vi "Point Turn.vi"(9 "Speed":dbl, 10 "Angle":dbl) -> ()   [LabVIEW 2019]
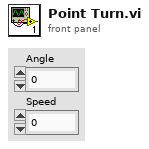
[diagram p1: front panel]
types:
  T1 = typedef "WPI_EncoderDevRef.ctl" = cluster{"DevStatus":errorcluster, "EncoderIndex":T2, "CounterIndex":T3, "DistancePerCount":dbl, "Decoding Type":T4}
  T2 = typedef "FPGA_EncoderIdx.ctl" = enum8{"Enc 0", "Enc 1", "Enc 2", "Enc 3", "Enc 4", "Enc 5", "Enc 6", "Enc 7", "Invalid"}
  T3 = typedef "FPGA_CounterCtrSystemIndex.ctl" = enum8{"Ctr 0", "Ctr 1", "Ctr 2", "Ctr 3", "Ctr 4", "Ctr 5", "Ctr 6", "Ctr 7", "Invalid"}
  T4 = typedef "WPI_EncoderType.ctl" = enum16{"1x", "2x", "4x"}
  T5 = typedef "WPI_RobotDriveDevRef.ctl" = cluster{"DevStatus":errorcluster, "Motors[]":T6[], "Square Inputs":bool, "Max Output":dbl}
  T6 = typedef "WPI_MotorControlDeviceRef.ctl" = cluster{"DeviceStatus":errorcluster, "Type":T7, "PWM":cluster{"PWM Channel":T8, "DeadBand":T9}, "CAN":cluster{"Device Number":u8, "SetOutput VI Ref":variant, "GetOutput VI Ref":variant, "Enable VI Ref":variant, "Disable VI Ref":variant, "Data":variant}, "Invert":bool, "DIO PWM":cluster{"PWM \"Enable\" Channel":T8, "DIOChannel":T10, "PWM Rate":dbl}}
  T7 = typedef "WPI_MotorControlType.ctl" = enum16{"PWM", "CAN", "DIO PWM"}
  T8 = typedef "FPGA_DIOPWMChannel.ctl" = enum8{"PWM 0", "PWM 1", "PWM 2", "PWM 3", "PWM 4", "PWM 5", "PWM 6", "PWM 7", "PWM 8", "PWM 9", "PWM MXP 0", "PWM MXP 1", "PWM MXP 2", "PWM MXP 3", "PWM MXP 4", "PWM MXP 5", "PWM MXP 6", "PWM MXP 7", "PWM MXP 8", "PWM MXP 9", "Invalid"}
  T9 = typedef "WPI_PWMDeadband.ctl" = cluster{"Name":string, "maxPositivePwm":i32, "minPositivePwm":i32, "centerPwm":i32, "maxNegativePwm":i32, "minNegativePwm":i32, "angularRange":u16}
  T10 = typedef "FPGA_DIOChannel.ctl" = enum8{"DIO 0", "DIO 1", "DIO 2", "DIO 3", "DIO 4", "DIO 5", "DIO 6", "DIO 7", "DIO 8", "DIO 9", "DIO MXP 0", "DIO MXP 1", "DIO MXP 2", "DIO MXP 3", "DIO MXP 4", "DIO MXP 5", "DIO MXP 6", "DIO MXP 7", "DIO MXP 8", "DIO MXP 9", "DIO MXP 10", "DIO MXP 11", "DIO MXP 12", "DIO MXP 13", "DIO MXP 14", "DIO MXP 15", "SPI Port CS1", "SPI Port CS2", "SPI Port CS3", "SPI Port MISO", "SPI Port MOSI", "Invalid"}
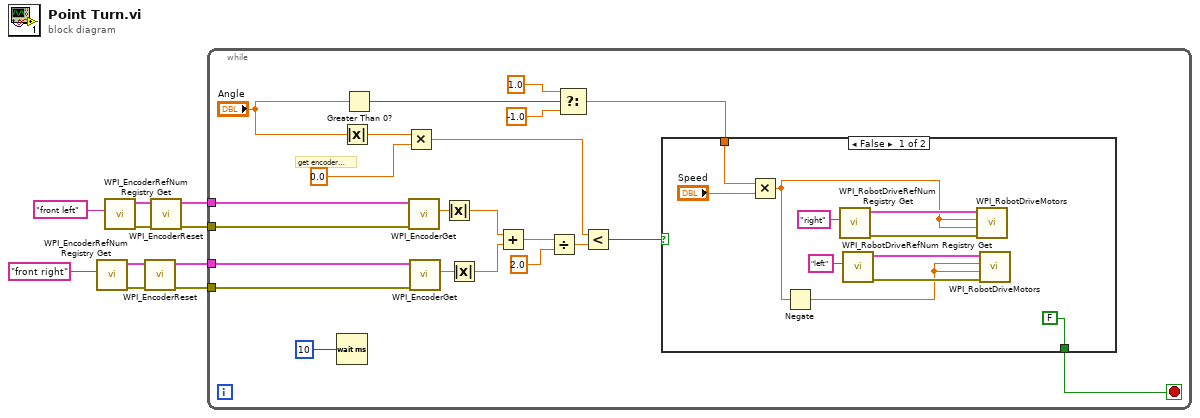
[diagram p0: block diagram]
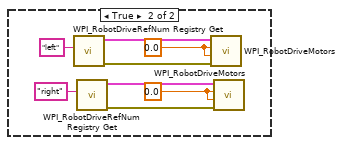
[diagram p2: hidden frame]
diagram:
  n1 = call <vilib>:"WPI_EncoderRefNum Registry Get.vi"("refnum name"="front right") -> ("error out"=w3:errorcluster, "EncoderDevRef"=w4:T1)  [unwired: 9 in]
  n2 = call <vilib>:"WPI_EncoderRefNum Registry Get.vi"("refnum name"="front left") -> ("error out"=w7:errorcluster, "EncoderDevRef"=w8:T1)  [unwired: 9 in]
  n3 = call <vilib>:"WPI_EncoderReset.vi"("error in (no error)"=w3, "EncoderDevRef"=w4) -> ("error out"=w1:errorcluster, "EncoderDevRef"=w2:T1)  [unwired: 8 in]
  n4 = call <vilib>:"WPI_EncoderReset.vi"("error in (no error)"=w7, "EncoderDevRef"=w8) -> ("error out"=w5:errorcluster, "EncoderDevRef"=w6:T1)  [unwired: 8 in]
  n5 = while {
    tunnel: w6 -> [w32]
    tunnel: w5 -> [w31]
    tunnel: w2 -> [w30]
    tunnel: w1 -> [w29]
    stop <- w11 stop-if-true
    # "get encoder ration"
    n6 = Wait (ms)(milliseconds to wait=u32 10 ("millisecond timer value")) -> ()  [unwired: 1 out]
    n7 = Absolute Value(x="Angle") -> (abs(x)=w19:dbl)
    n8 = Greater Than 0?(x="Angle") -> (x > 0?=w18:bool)
    n9 = Multiply(x=w19, y=0.0) -> (x*y=w20:dbl)
    n10 = call <vilib>:"WPI_EncoderGet.vi"("error in (no error)"=w31, "EncoderDevRef"=w32) -> ("Distance"=w27:dbl)  [unwired: 4 in, 5 out]
    n11 = call <vilib>:"WPI_EncoderGet.vi"("error in (no error)"=w29, "EncoderDevRef"=w30) -> ("Distance"=w28:dbl)  [unwired: 4 in, 5 out]
    n12 = Absolute Value(x=w27) -> (abs(x)=w26:dbl)
    n13 = Absolute Value(x=w28) -> (abs(x)=w25:dbl)
    n14 = Add(x=w26, y=w25) -> (x+y=w24:dbl)
    n15 = Divide(x=w24, y=2.0) -> (x/y=w22:dbl)
    n16 = Select(t=1.0, s=w18, f=-1.0) -> (s? t:f=w14:dbl)
    n17 = Less?(x=w20, y=w22) -> (x < y?=w15:bool)
    n18 = case shown="False" w15 {
      tunnel: w14 -> [w37 _]
      tunnel: [FALSE _] -> w11
      frame False {
        n19 = Multiply(x=w37, y="Speed") -> (x*y=w34:dbl)
        n20 = Negate(x=w34) -> (-x=w35:dbl)
        n21 = call <vilib>:"WPI_RobotDriveRefNum Registry Get.vi"("refnum name"="right") -> ("error out"=w41:errorcluster, "RobotDriveDevRef"=w40:T5)  [unwired: 9 in]
        n22 = call <vilib>:"WPI_RobotDriveRefNum Registry Get.vi"("refnum name"="left") -> ("error out"=w43:errorcluster, "RobotDriveDevRef"=w42:T5)  [unwired: 9 in]
        n23 = call <vilib>:"WPI_RobotDriveMotors.vi"("error in (no error)"=w41, "RightSpeed"=w34, "LeftSpeed"=w34, "RobotDriveDevRef"=w40) -> ()  [unwired: 5 in, 3 out]
        n24 = call <vilib>:"WPI_RobotDriveMotors.vi"("error in (no error)"=w43, "RightSpeed"=w35, "LeftSpeed"=w35, "RobotDriveDevRef"=w42) -> ()  [unwired: 5 in, 3 out]
      }
      frame True {
        w44 = 0.0 ("LeftSpeed")
        w45 = 0.0 ("LeftSpeed")
        n25 = call <vilib>:"WPI_RobotDriveRefNum Registry Get.vi"("refnum name"="left") -> ("error out"=w50:errorcluster, "RobotDriveDevRef"=w51:T5)  [unwired: 9 in]
        n26 = call <vilib>:"WPI_RobotDriveRefNum Registry Get.vi"("refnum name"="right") -> ("error out"=w47:errorcluster, "RobotDriveDevRef"=w48:T5)  [unwired: 9 in]
        n27 = call <vilib>:"WPI_RobotDriveMotors.vi"("error in (no error)"=w50, "RightSpeed"=w45, "LeftSpeed"=w45, "RobotDriveDevRef"=w51) -> ()  [unwired: 5 in, 3 out]
        n28 = call <vilib>:"WPI_RobotDriveMotors.vi"("error in (no error)"=w47, "RightSpeed"=w44, "LeftSpeed"=w44, "RobotDriveDevRef"=w48) -> ()  [unwired: 5 in, 3 out]
      }
    }
  }
